vi "Recursive File List2.vi"(8 "error in (no error)":errorcluster, 10 "patterns":string[](array[string])=["*.py"], 11 "Folder Path":path) -> (0 "error out":errorcluster, 2 "All Files in Dir":path[](array[path]), 3 "dup Folder Path":path)   [LabVIEW 2022 SP3]
doc: "Lists the contents of a folder or LLB. In order for this VI to work correctly, the LLB must have a .llb file extension."
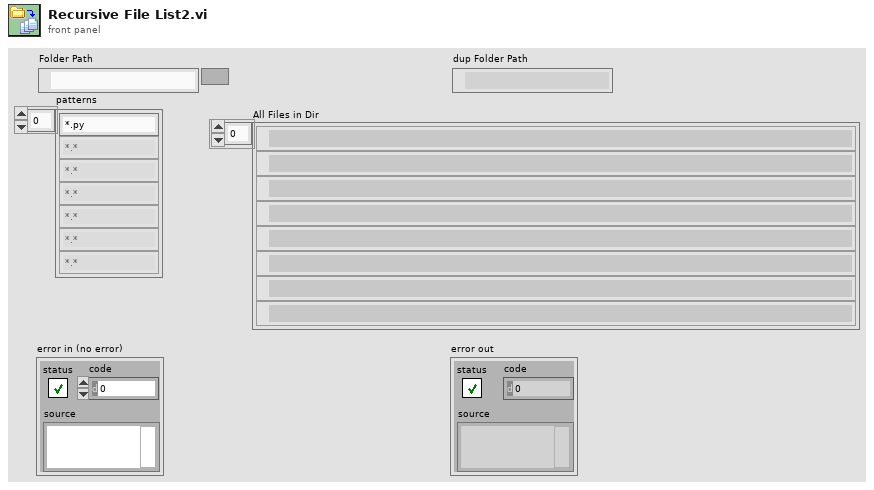
[diagram p1: front panel]
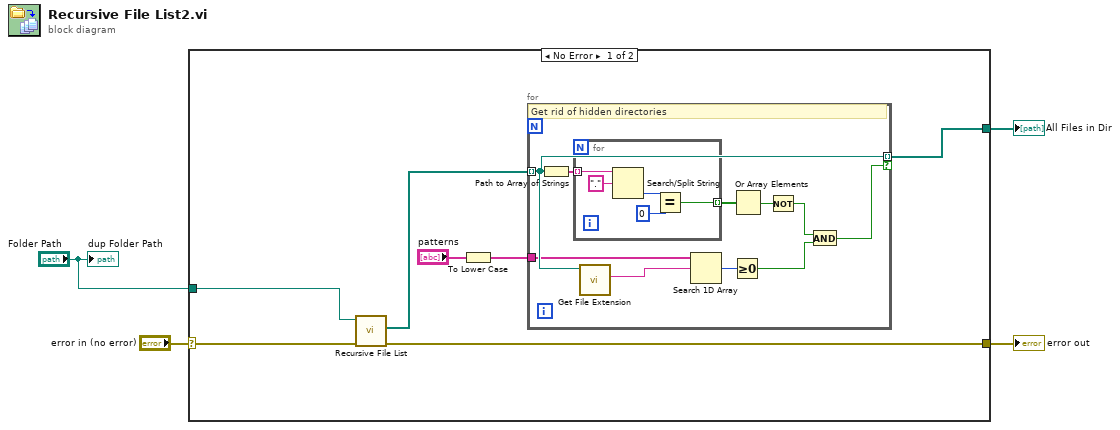
[diagram p0: block diagram]
diagram:
  n1 = case shown="No Error" "error in (no error)" {
    selector: "error in (no error)" -> [w10 w27]
    tunnel: "Folder Path" -> [w11 _]
    tunnel: [w8 _] -> w4
    tunnel: [w9 w27] -> w3
    frame No Error {
      n2 = call <vilib>:"Recursive File List.vi"("error in (no error)"=w10, "Folder Path"=w11) -> ("error out"=w9:errorcluster, "All Files in Dir"=w5:path[])  [unwired: 5 in, 3 out]
      n3 = To Lower Case(string="patterns") -> (all lower case string=w6:string[])
      n4 = for {
        tunnel: w5 -> [w18] mode=indexing
        tunnel: [w18] -> w8 mode=indexing if=w12
        tunnel: w6 -> [w17]
        # "Get rid of hidden directories"
        n5 = Path to Array of Strings(0:w18) -> (2:w21:string[])  [unwired: 1 out]
        n6 = for {
          tunnel: w21 -> [w26] mode=indexing
          tunnel: [w22] -> w20 mode=indexing
          n7 = Search/Split String(string=w26, search string/char (-)=".") -> (offset of match=w24:i32)  [unwired: 1 in, 2 out]
          n8 = Equal?(x=w24, y=0) -> (x = y?=w22:bool)
        }
        n9 = call <vilib>:"Get File Extension.vi"("file"=w18) -> ("lowercase file extension"=w16:string)  [unwired: 6 in, 4 out]
        n10 = Search 1D Array(1D array=w17, element=w16) -> (index of element=w15:i32)  [unwired: 1 in]
        n11 = Greater Or Equal To 0?(x=w15) -> (x >= 0?=w13:bool)
        n12 = Or Array Elements(Boolean array=w20) -> (logical OR=w19:bool)
        n13 = Not(x=w19) -> (.not. x?=w14:bool)
        n14 = And(x=w14, y=w13) -> (x .and. y?=w12:bool)
      }
    }
    frame Error {
    }
  }
  "All Files in Dir" <- w4
  "error out" <- w3
  "dup Folder Path" <- "Folder Path"
